vi "PopUp Chart.vi"() -> ()   [LabVIEW 2016, in "Display Panel.lvlib" / "Universal Display.lvclass"]
uses:
  Universal Display.lvclass
panel:
  out "Pages":refnum<vi>[](array[refnum])
  in  "Tab Control":enum32{"Page 1", "Page 2", "Page 3"}(tab)
  out "Waveform Chart":dbl(graph)
  out "Waveform Chart  2":dbl(graph)
  out "Waveform Chart  3":dbl(graph)
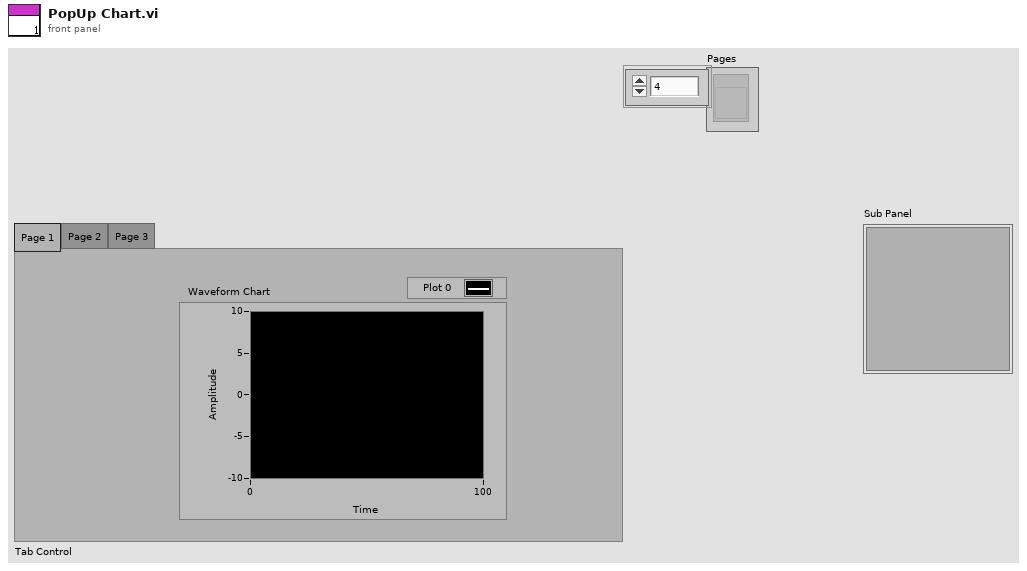
[diagram p1: front panel]
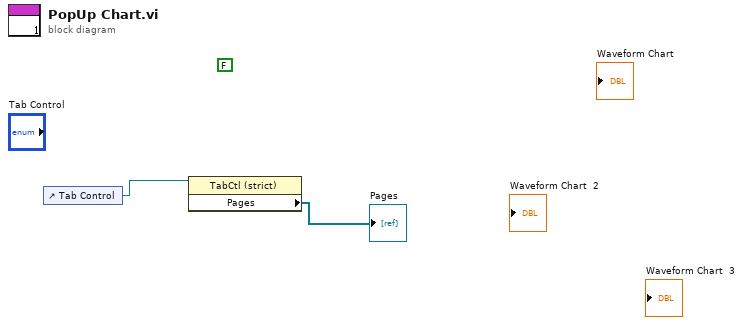
[diagram p0: block diagram]
diagram:
  (unwired) FALSE ("Indicator")
  n1 = control-ref of="Tab Control"() -> (w2:refnum<vi>)
  n2 = property class="TabCtl (strict)"(reference=w2) -> ("Pages"=→"Pages":refnum<vi>[])  [unwired: 1 in, 2 out]
